vi "ClearCache.vi"   [LabVIEW 2015]
uses:
  <vilib>/Wiresmith Technology/G CLI/CLI Class/CLI.lvclass
panel:
  # "Clear Caches...."
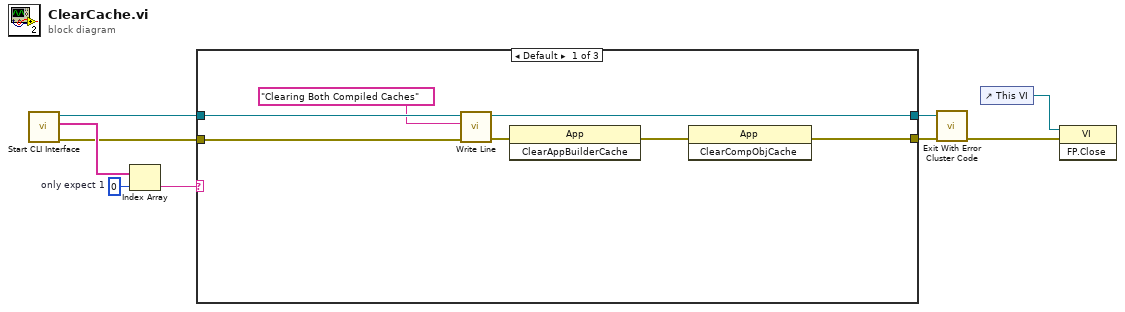
[diagram p0: block diagram]
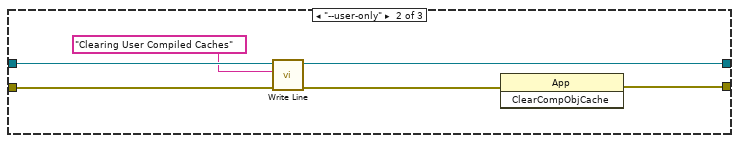
[diagram p2: hidden frame]
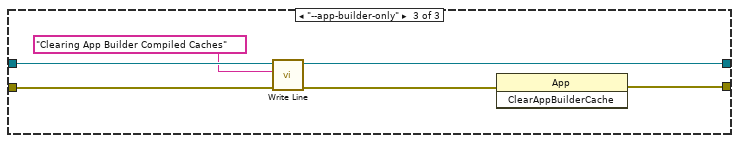
[diagram p3: hidden frame]
diagram:
  w8 = 0  # only expect 1
  n1 = call <vilib>:"Start CLI Interface.vi"() -> ("error out"=w5:errorcluster, "Custom Parameters"=w9:string[], "CLI out"=w6:refnum<class "CLI.lvclass">)  [unwired: 8 in, 1 out]
  n2 = Index Array(array=w9, index=w8) -> (element=w7:string)
  n3 = case shown="Default" w7 {
    tunnel: w6 -> [w16 w22 w28]
    tunnel: w5 -> [w15 w21 w27]
    tunnel: [w11 w18 w24] -> w4
    tunnel: [w10 w17 w23] -> w3
    frame Default {
      n4 = call <vilib>:"Write Line.vi"("error in (no error)"=w15, "Text to Write"="Clearing Both Compiled Caches", "CLI in"=w16) -> ("error out"=w13:errorcluster, "CLI out"=w10:refnum<class "CLI.lvclass">)  [unwired: 7 in]
      n5 = invoke class="App" method="ClearAppBuilderCache"(error in=w13) -> (error out=w12:errorcluster)  [unwired: 2 in, 2 out]
      n6 = invoke class="App" method="ClearCompObjCache"(error in=w12) -> (error out=w11:errorcluster)  [unwired: 2 in, 2 out]
    }
    frame "--user-only" {
      n7 = call <vilib>:"Write Line.vi"("error in (no error)"=w21, "Text to Write"="Clearing User Compiled Caches", "CLI in"=w22) -> ("error out"=w19:errorcluster, "CLI out"=w17:refnum<class "CLI.lvclass">)  [unwired: 7 in]
      n8 = invoke class="App" method="ClearCompObjCache"(error in=w19) -> (error out=w18:errorcluster)  [unwired: 2 in, 2 out]
    }
    frame "--app-builder-only" {
      n9 = call <vilib>:"Write Line.vi"("error in (no error)"=w27, "Text to Write"="Clearing App Builder Compiled Caches", "CLI in"=w28) -> ("error out"=w25:errorcluster, "CLI out"=w23:refnum<class "CLI.lvclass">)  [unwired: 7 in]
      n10 = invoke class="App" method="ClearAppBuilderCache"(error in=w25) -> (error out=w24:errorcluster)  [unwired: 2 in, 2 out]
    }
  }
  n11 = call <vilib>:"Exit With Error Cluster Code.vi"("error in (no error)"=w4, "CLI in"=w3) -> ("error out"=w1:errorcluster)  [unwired: 9 in]
  n12 = control-ref of="This VI"() -> (w2:refnum<vi>)
  n13 = invoke class="VI" method="FP.Close"(reference=w2, error in=w1) -> ()  [unwired: 1 in, 3 out]
